vi "take_spectrum.vi"() -> ()   [LabVIEW 2018]
uses:
  <vilib>/Utility/file.llb/Write Delimited Spreadsheet (DBL).vi
panel:
  in  "Resume":bool
  out "Error Out":errorcluster
  in  "Scan Name":string
  in  "Scan Directory":string="Peter_ferguson\\test_scans\\Tcal Labview\\"
  in  "Integration time":dbl
  out "Spectrometer":cluster{"Y":dbl[], "Y":dbl[]}[](graph)
  out "Number of Spectrometers":i32
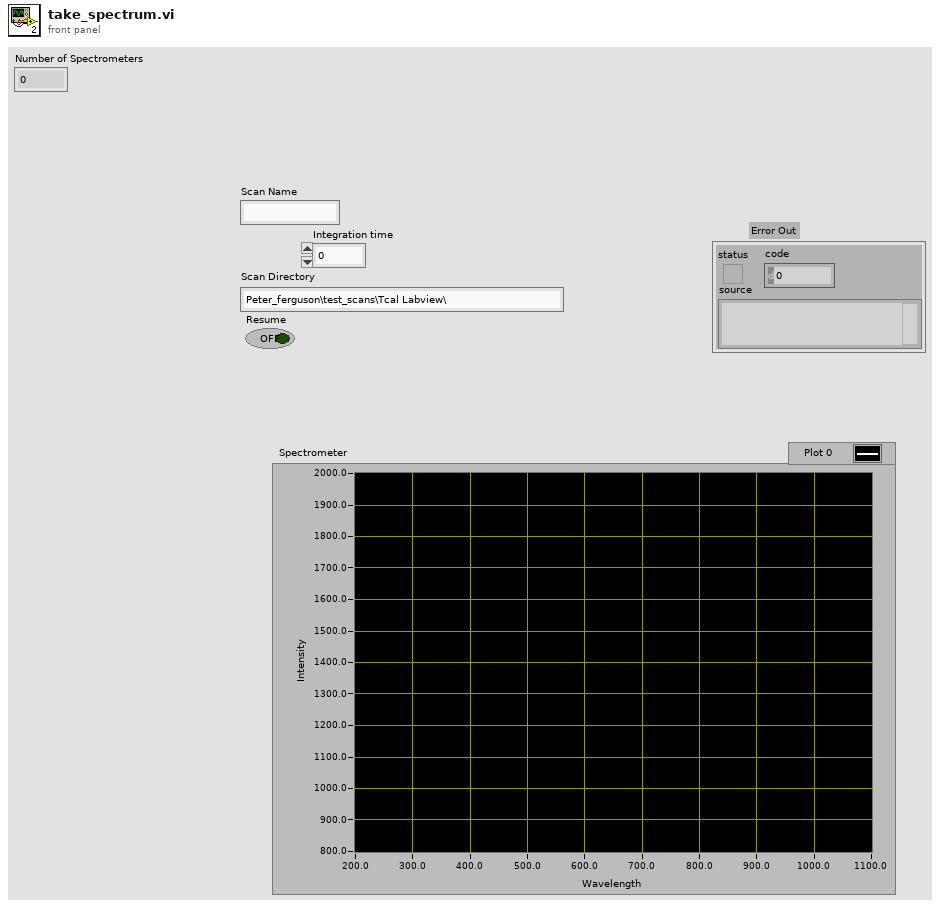
[diagram p1: front panel]
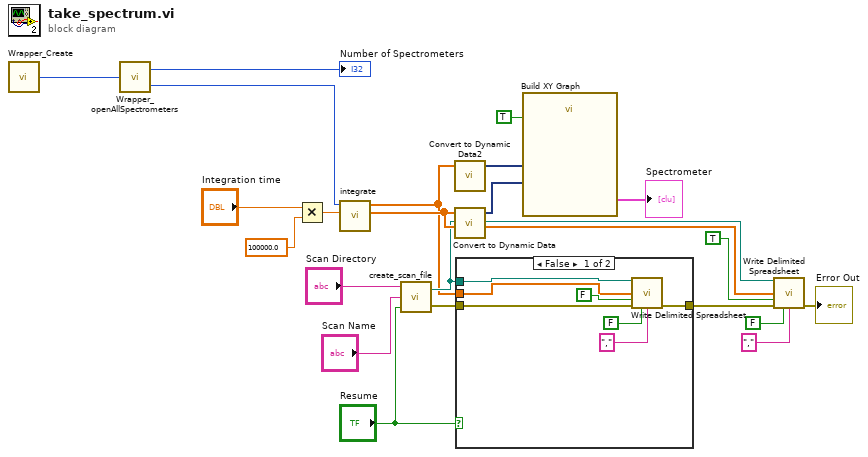
[diagram p0: block diagram]
diagram:
  n1 = call "Wrapper_Create.vi"() -> ("Wrapper"=w18:u64)
  n2 = call "Wrapper_openAllSpectrometers.vi"("Wrapper In"=w18) -> ("Number of Spectrometers"=→"Number of Spectrometers":i32, "Wrapper Out"=w16:u64)
  n3 = Multiply(x="Integration time", y=100000.0) -> (x*y=w15:dbl)
  n4 = call "integrate.vi"("Numeric"=w15, "Wrapper Out"=w16) -> ("Spectrum Values"=w11:dbl[], "WL Values"=w3:dbl[])  [unwired: 7 in, 1 out]
  n5 = call "create_scan_file.vi"("Resume"="Resume", "Scan Name"="Scan Name", "Scan Directory"="Scan Directory") -> ("Error Out"=w6:errorcluster, "path"=w4:path)
  n6 = call "Convert to Dynamic Data2"("Array"=w3) -> ("Dynamic Data Type"=w21:dynamicdata)  [unwired: 3 in]
  n7 = call "Convert to Dynamic Data"("Array"=w11) -> ("Dynamic Data Type"=w22:dynamicdata)  [unwired: 3 in]
  n8 = case shown="False" "Resume" {
    tunnel: w6 -> [w26 w30]
    tunnel: [w25 w30] -> w5
    tunnel: w4 -> [w24 _]
    tunnel: w3 -> [w23 _]
    frame False {
      n9 = call-poly <vilib>:"Write Delimited Spreadsheet.vi"("file path (dialog if empty)"=w24, "1D data"=w23, "append to file? (new file:F)"=FALSE, "error in (no error)"=w26, "transpose? (no:F)"=FALSE, "delimiter (\\t)"="," ("delimiter (\\t)")) -> ("error out"=w25:errorcluster)  [unwired: 8 in, 1 out]
    }
    frame True {
    }
  }
  n10 = call "Build XY Graph"("Reset"=TRUE, "Y Input"=w22, "X Input"=w21) -> ("XY Graph"=→"Spectrometer":cluster{"X":dbl[], "Y":dbl[]}[])  [unwired: 7 in, 1 out]
  n11 = call-poly <vilib>:"Write Delimited Spreadsheet.vi"("file path (dialog if empty)"=w4, "1D data"=w11, "append to file? (new file:F)"=TRUE, "error in (no error)"=w5, "transpose? (no:F)"=FALSE, "delimiter (\\t)"="," ("delimiter (\\t)")) -> ("error out"=→"Error Out":errorcluster)  [unwired: 8 in, 1 out]
